vi "convert.vi"(8 "error in (no error)":errorcluster, 10 "Input":dbl, 11 "IConverterStrategy in":refnum<class "IConverterStrategy.lvclass">) -> (0 "error out":errorcluster, 2 "Output":dbl, 3 "IConverterStrategy out":refnum<class "IConverterStrategy.lvclass">)   [LabVIEW 2015, in "IConverterStrategy.lvclass"]
uses:
  IConverterStrategy.lvclass
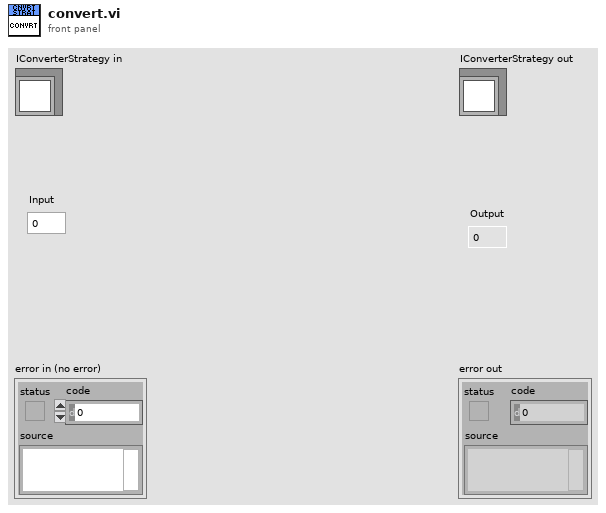
[diagram p1: front panel]
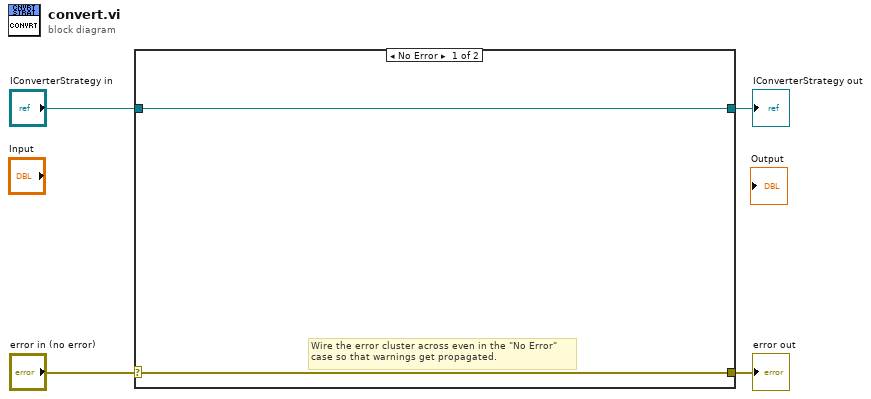
[diagram p0: block diagram]
diagram:
  n1 = case shown="No Error" "error in (no error)" {
    selector: "error in (no error)" -> [w5 w8]
    tunnel: [w5 w8] -> w3
    tunnel: [w6 w7] -> w1
    tunnel: "IConverterStrategy in" -> [w6 w7]
    frame No Error {
      # "Wire the error cluster across even in the \"No Error\"\ncase so that warnings get propagated."
    }
    frame Error {
    }
  }
  "error out" <- w3
  "IConverterStrategy out" <- w1
